vi "FPGA_trigger_camera_synchro_laser_lines_v0.vi"(2 "Trigger type":i16(ring) items=["UP is ready", "DOWN is ready"], 3 "N images":i32) -> ()   [LabVIEW 2015]
uses:
  <vilib>/rvi/Emulation/niFpgaGetClockAttributes.vi
  <vilib>/rvi/Emulation/niFpgaSctlEmulationGetInTimedLoop.vi
  <vilib>/rvi/Emulation/niFpgaEmulationReportErrorSimple.vi
  <vilib>/rvi/eio/common/nirviEmuTemplateMethod_errors.vi
  <vilib>/rvi/Emulation/niFpgaCriticalErrorInLSC.vi
  <vilib>/eio/EIONode/EIONode.xnode
panel:
  in  "Trigger count(uSec)":u32 caption="Count(uSec)"
  out "Images acquired":i32
  in  "Laser lines":i32[](array[numeric])=[0, 0, 0, 0, 0]
  in  "Laser power":sgl[](array[numeric])=[0.0, 0.0, 0.0, 0.0, 0.0]
  in  "N laser lines":i32
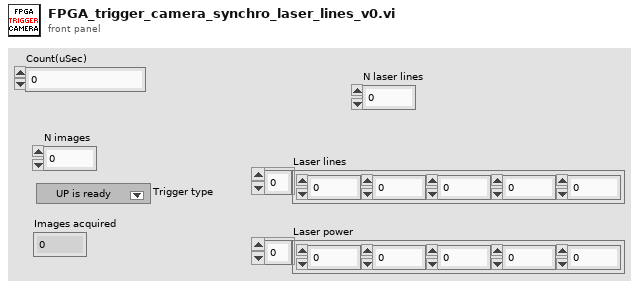
[diagram p1: front panel]
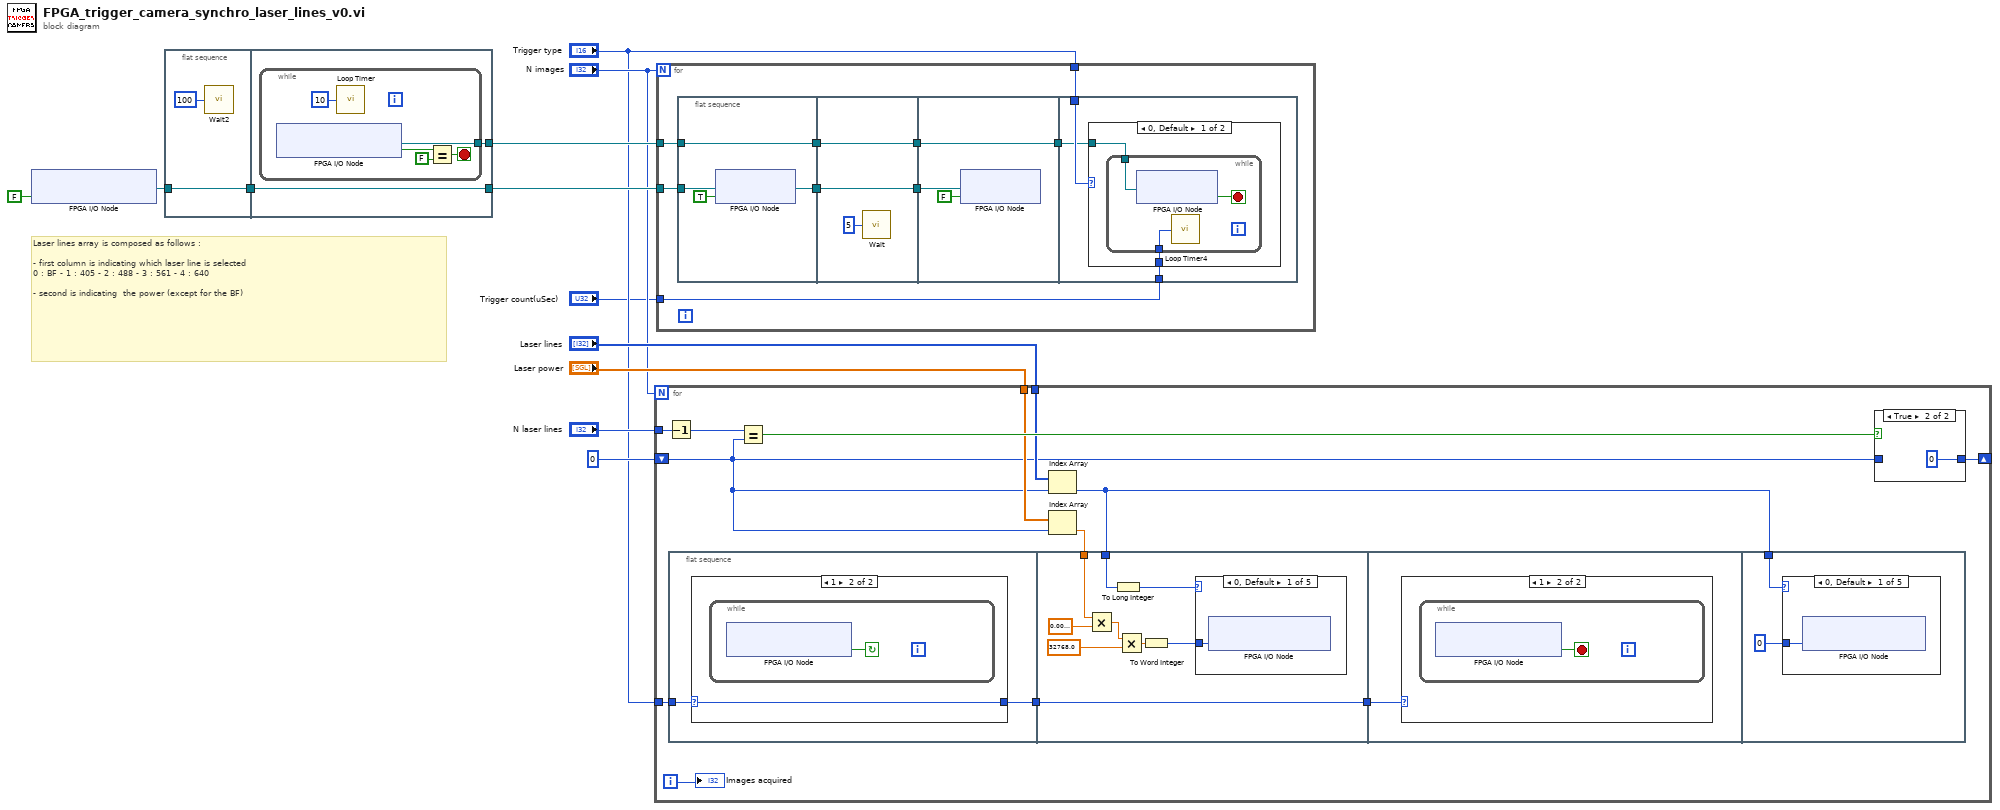
[diagram p0: block diagram]
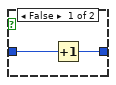
[diagram p2: hidden frame]
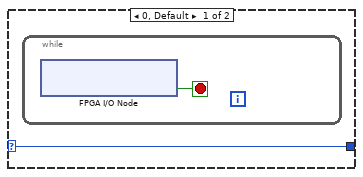
[diagram p3: hidden frame]
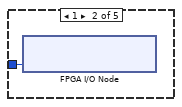
[diagram p4: hidden frame]
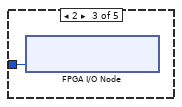
[diagram p5: hidden frame]
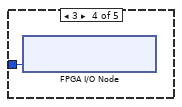
[diagram p6: hidden frame]
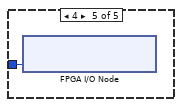
[diagram p7: hidden frame]
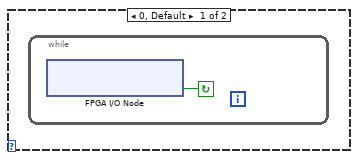
[diagram p8: hidden frame]
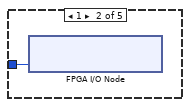
[diagram p9: hidden frame]
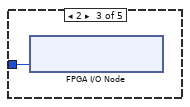
[diagram p10: hidden frame]
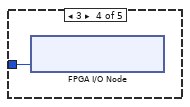
[diagram p11: hidden frame]
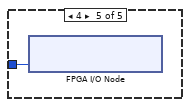
[diagram p12: hidden frame]
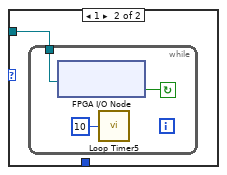
[diagram p13: hidden frame]
diagram:
  # "Laser lines array is composed as follows :\n\n- first column is indicating which laser line is selected \n0 : BF - 1 : 405 - 2 : 488 - 3 : 561 - 4 : 640\n\n- second is indicating  the power (except for the BF)"
  n1 = xnode "FPGA I/O Node"("Connector0/DIO0"=FALSE) -> ("FPGA I/O Out"=w11:refnum<k21>)  [unwired: 1 in]
  n2 = flat-sequence {
    tunnel: w11 -> [w14]
    tunnel: [w14] -> w10
    tunnel: w10 -> [w16]
    tunnel: [w16] -> w9
    tunnel: [w15] -> w8
    frame #0 {
      n3 = call "Wait2"("Count(uSec)"=u32 100 ("Count(mSec)")) -> ()  [unwired: 1 out]
    }
    frame #1 {
      n4 = while {
        tunnel: [w21] -> w15
        stop <- w17 stop-if-true
        n5 = xnode "FPGA I/O Node"() -> ("Connector0/DIO1"=w19:bool, "FPGA I/O Out"=w21:refnum<k21>)  [unwired: 1 in]
        n6 = call "Loop Timer"("Count(uSec)"=u32 10) -> ()  [unwired: 1 out]
        n7 = Equal?(x=w19, y=FALSE) -> (x = y?=w17:bool)
      }
    }
  }
  n8 = for {
    N: "N images" -> [_]
    tunnel: "Trigger type" -> [w34]
    shift-right: [w29] -> _
    shift-left: 0 -> [w26]
    tunnel: "Laser lines" -> [w28]
    tunnel: "Laser power" -> [w27]
    tunnel: "N laser lines" -> [w24]
    i -> [w22]
    n9 = Decrement(x=w24) -> (x-1=w23:i32)
    n10 = flat-sequence {
      tunnel: w34 -> [w39]
      tunnel: [w38] -> w33
      tunnel: w31 -> [w46]
      tunnel: w33 -> [w47]
      tunnel: [w47] -> w32
      tunnel: w25 -> [w45]
      tunnel: w32 -> [w58]
      tunnel: w31 -> [w61]
      frame #0 {
        n11 = case shown="1" w39 {
          selector: w39 -> [w40 w42]
          tunnel: [w40 w42] -> w38
          frame 0, Default {
            n12 = while {
              stop <- w41 stop-if-true
              n13 = xnode "FPGA I/O Node"() -> ("Connector0/DIO2"=w41:bool)  [unwired: 1 in, 1 out]
            }
          }
          frame 1 {
            n14 = while {
              stop <- w43 continue-if-true
              n15 = xnode "FPGA I/O Node"() -> ("Connector0/DIO2"=w43:bool)  [unwired: 1 in, 1 out]
            }
          }
        }
      }
      frame #1 {
        n16 = Multiply(x=w45, y=sgl 0.01) -> (x*y=w44:sgl)
        n17 = To Long Integer(number=w46) -> (32bit integer=w52:i32)
        n18 = Multiply(x=w44, y=sgl 32768.0) -> (x*y=w49:sgl)
        n19 = To Word Integer(number=w49) -> (16bit integer=w48:i16)
        n20 = case shown="0, Default" w52 {
          tunnel: w48 -> [w53 w54 w55 w56 w57]
          frame 0, Default {
            n21 = xnode "FPGA I/O Node"("Connector0/AO0"=w53) -> ()  [unwired: 1 in, 1 out]
          }
          frame 1 {
            n22 = xnode "FPGA I/O Node"("Connector0/AO0"=w54) -> ()  [unwired: 1 in, 1 out]
          }
          frame 2 {
            n23 = xnode "FPGA I/O Node"("Connector0/AO0"=w55) -> ()  [unwired: 1 in, 1 out]
          }
          frame 3 {
            n24 = xnode "FPGA I/O Node"("Connector0/AO0"=w56) -> ()  [unwired: 1 in, 1 out]
          }
          frame 4 {
            n25 = xnode "FPGA I/O Node"("Connector0/AO0"=w57) -> ()  [unwired: 1 in, 1 out]
          }
        }
      }
      frame #2 {
        n26 = case shown="1" w58 {
          frame 0, Default {
            n27 = while {
              stop <- w59 continue-if-true
              n28 = xnode "FPGA I/O Node"() -> ("Connector0/DIO2"=w59:bool)  [unwired: 1 in, 1 out]
            }
          }
          frame 1 {
            n29 = while {
              stop <- w60 stop-if-true
              n30 = xnode "FPGA I/O Node"() -> ("Connector0/DIO2"=w60:bool)  [unwired: 1 in, 1 out]
            }
          }
        }
      }
      frame #3 {
        n31 = case shown="0, Default" w61 {
          tunnel: i16 0 -> [w63 w64 w65 w66 w67]
          frame 0, Default {
            n32 = xnode "FPGA I/O Node"("Connector0/AO0"=w63) -> ()  [unwired: 1 in, 1 out]
          }
          frame 1 {
            n33 = xnode "FPGA I/O Node"("Connector0/AO0"=w64) -> ()  [unwired: 1 in, 1 out]
          }
          frame 2 {
            n34 = xnode "FPGA I/O Node"("Connector0/AO0"=w65) -> ()  [unwired: 1 in, 1 out]
          }
          frame 3 {
            n35 = xnode "FPGA I/O Node"("Connector0/AO0"=w66) -> ()  [unwired: 1 in, 1 out]
          }
          frame 4 {
            n36 = xnode "FPGA I/O Node"("Connector0/AO0"=w67) -> ()  [unwired: 1 in, 1 out]
          }
        }
      }
    }
    n37 = Equal?(x=w23, y=w26) -> (x = y?=w30:bool)
    n38 = Index Array(array=w28, index=w26) -> (element=w31:i32)
    n39 = Index Array(array=w27, index=w26) -> (element=w25:sgl)
    n40 = case shown="True" w30 {
      tunnel: w26 -> [w36 _]
      tunnel: [w35 0] -> w29
      frame False {
        n41 = Increment(x=w36) -> (x+1=w35:i32)
      }
      frame True {
      }
    }
    "Images acquired" <- w22
  }
  n42 = for {
    N: "N images" -> [_]
    tunnel: w9 -> [w74]
    tunnel: "Trigger type" -> [w73]
    tunnel: w8 -> [w72]
    tunnel: "Trigger count(uSec)" -> [w68]
    n43 = flat-sequence {
      tunnel: [w79] -> w76
      tunnel: w74 -> [w78]
      tunnel: w72 -> [w77]
      tunnel: [w77] -> w69
      tunnel: w76 -> [w82]
      tunnel: [w82] -> w75
      tunnel: [w81] -> w70
      tunnel: w69 -> [w81]
      tunnel: w75 -> [w85]
      tunnel: [w84] -> w71
      tunnel: w70 -> [w84]
      tunnel: w73 -> [w89]
      tunnel: w71 -> [w88]
      tunnel: w68 -> [w87]
      frame #0 {
        n44 = xnode "FPGA I/O Node"("I/O Item"=TRUE ("Connector0/DIO0"), "FPGA I/O In"=w78) -> ("FPGA I/O Out"=w79:refnum<k21>)
      }
      frame #1 {
        n45 = call "Wait"("Count(mSec)"=u32 5) -> ()  [unwired: 1 out]
      }
      frame #2 {
        n46 = xnode "FPGA I/O Node"("I/O Item"=FALSE ("Connector0/DIO0"), "FPGA I/O In"=w85) -> ()  [unwired: 1 out]
      }
      frame #3 {
        n47 = case shown="0, Default" w89 {
          tunnel: w88 -> [w91 w95]
          tunnel: w87 -> [w90 _]
          frame 0, Default {
            n48 = while {
              tunnel: w91 -> [w94]
              tunnel: w90 -> [w92]
              stop <- w93 stop-if-true
              n49 = xnode "FPGA I/O Node"("FPGA I/O In"=w94) -> ("I/O Item"=w93:bool)  [unwired: 1 out]
              n50 = call "Loop Timer4"("Count(uSec)"=w92) -> ()  [unwired: 1 out]
            }
          }
          frame 1 {
            n51 = while {
              tunnel: w95 -> [w98]
              stop <- w96 continue-if-true
              n52 = xnode "FPGA I/O Node"("FPGA I/O In"=w98) -> ("I/O Item"=w96:bool)  [unwired: 1 out]
              n53 = call "Loop Timer5"("Count(uSec)"=u32 10) -> ()  [unwired: 1 out]
            }
          }
        }
      }
    }
  }
